vi "Enqueue--config_buttons.vi"(8 "error in (no error)":errorcluster, 11 "config_buttons":T1) -> (0 "error out":errorcluster)   [LabVIEW 2020, in "main.lvlib"]
doc: "Blank VI with error handling."
uses:
  main.lvlib
  config_buttons--enum.ctl
panel:
  # "Development\ncontrols/indicators useful for development and testing, but which are not outputs of the VI"
  # "Input\nInputs to the VI"
  # "Output\nOutputs of the VI"
  # "Description\n\nBlank VI with error handling case. \n\nSummarize the use of this VI in this space."
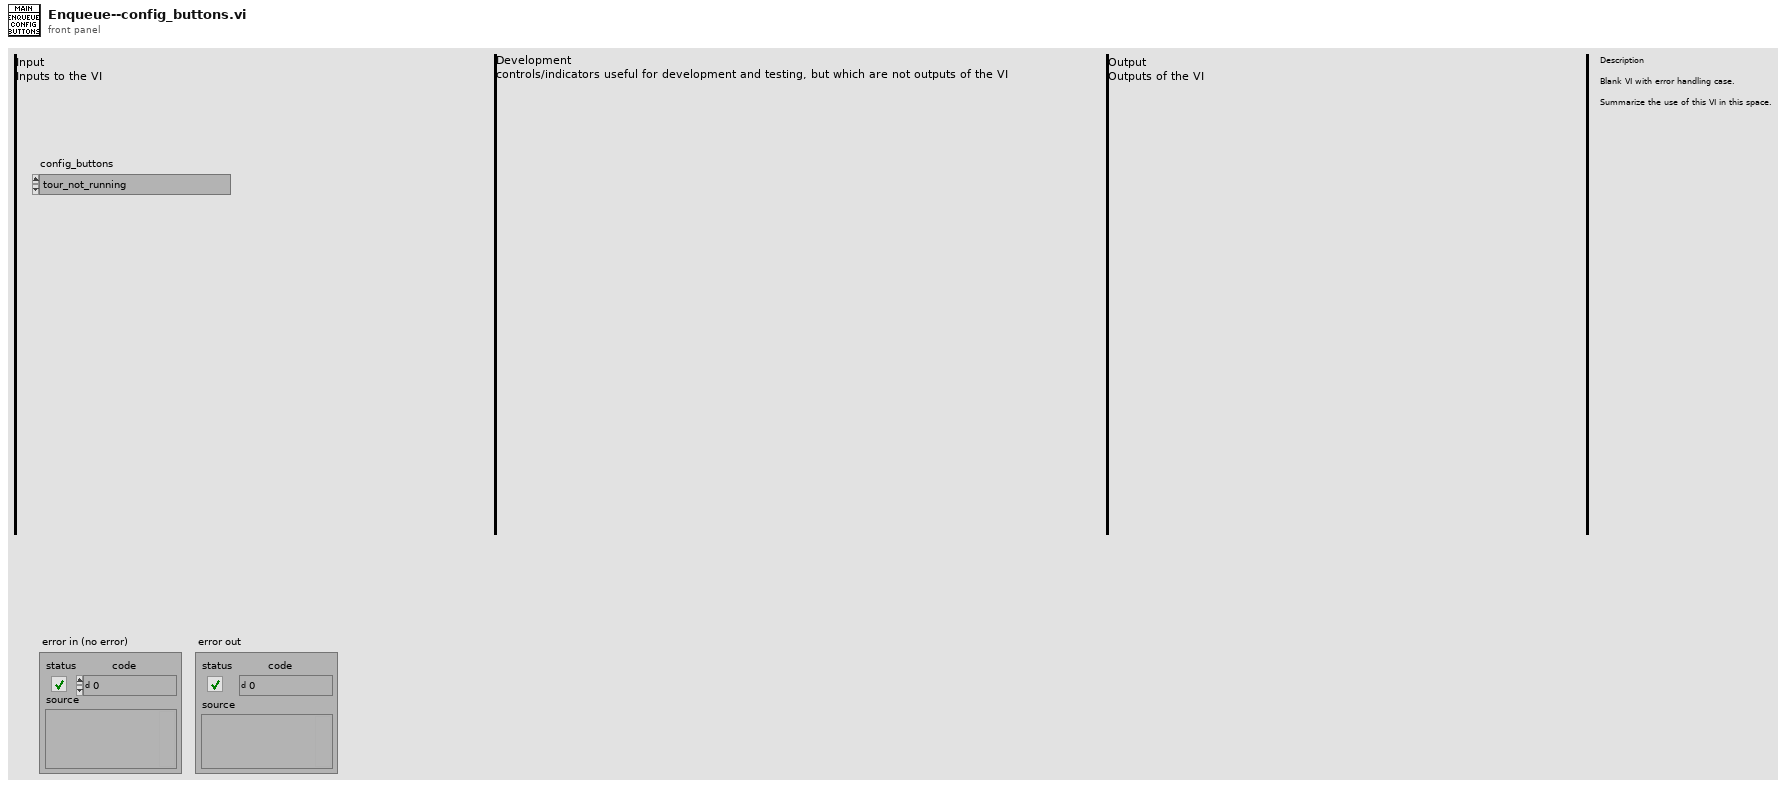
[diagram p1: front panel]
types:
  T1 = typedef "main.lvlib/config_buttons--enum.ctl" = enum16{"tour_not_running", "tour_running", "tour_paused"}
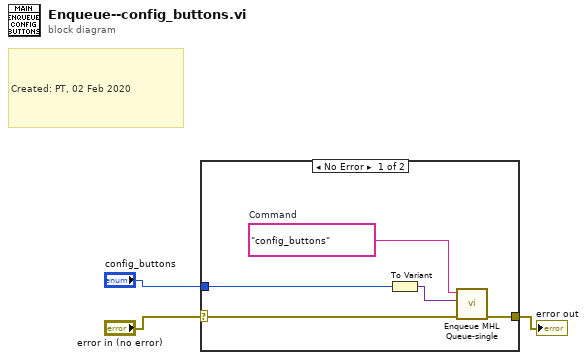
[diagram p0: block diagram]
diagram:
  # "Created: PT, 02 Feb 2020"
  n1 = case shown="No Error" "error in (no error)" {
    selector: "error in (no error)" -> [w7 w9]
    tunnel: [w6 w9] -> w2
    tunnel: "config_buttons" -> [w4 _]
    frame No Error {
      w8 = "config_buttons"  # Command
      n2 = To Variant(anything=w4) -> (Variant=w5:variant)
      n3 = call "Enqueue MHL Queue-single.vi"("ErrorIn"=w7, "Data"=w5, "Command"=w8) -> ("ErrorOut"=w6:errorcluster)  [unwired: 8 in]
    }
    frame Error {
    }
  }
  "error out" <- w2
